vi "Turbo Pump Control.vi"(8 "error in (no error)":errorcluster, 11 "cRIO-CO2 in":refnum<class "cRIO-CO2.lvclass">) -> ()   [LabVIEW 2015, in "cRIO-Carbondioxide.lvlib" / "cRIO-CO2.lvlib" / "cRIO-CO2.lvclass"]
uses:
  cRIO-CO2.lvclass
  <instrlib>/BOC Edwards TIC/Turbo Instrument Controller.llb/Type Def - Pump State.ctl
  <instrlib>/BOC Edwards TIC/Turbo Instrument Controller.llb/Type Def - Alert ID.ctl
  <instrlib>/BOC Edwards TIC/Turbo Instrument Controller.llb/Type Def - Priority.ctl
  Controls/Pumping State Enumerator.ctl
panel:
  in  "Running Dt":i32=1000
  out "Alert Priority":T1
  out "Status":T2
  out "Turbo Pump State":T3
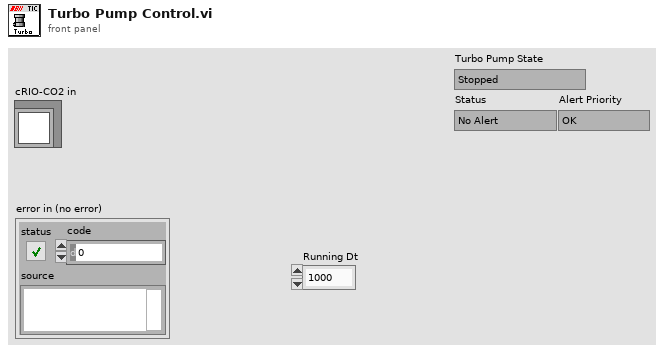
[diagram p1: front panel]
types:
  T1 = typedef "Type Def - Priority.ctl" = enum16{"OK", "Warning", "Alarm"}
  T2 = typedef "Type Def - Alert ID.ctl" = enum16{"No Alert", "ADC Fault", "ADC Not Ready", "Over Range", "Under Range", "ADC Invalid", "No Gauge", "Unknown", "Not Supported", "New ID", "Ion EM Timeout", "Not Struck", "Filament Fail", "Mag Fail", "Striker Fail", "Cal Error", "Initialising", "Emission Error", "Over Pressure", "ASG Can't Zero", "Ramp Up Timeout", "Droop Timeout", "Run Hours High", "SC Interlock", "ID Volts Error", "Serial ID Fail", "Upload Active", "DX Fault", "Temp Alert", "SYSI Inhibit", "Ext Inhibit", "Temp Inhibit", "No Reading", "No Message", "NOV Failure", "ULoad Timeout", "DLoad Failed", "No Tube"}
  T3 = typedef "Type Def - Pump State.ctl" = enum16{"Stopped", "Starting Delay", "Stopping Short Delay", "Stopping Normal Delay", "Running", "Accelerating", "Fault Braking", "Braking"}
  T4 = typedef "Pumping State Enumerator.ctl" = enum16{"Initialize", "Idle", "Error", "Start FV Pump", "Wait on FV Gauge", "Start Turbo", "Running", "Stop"}
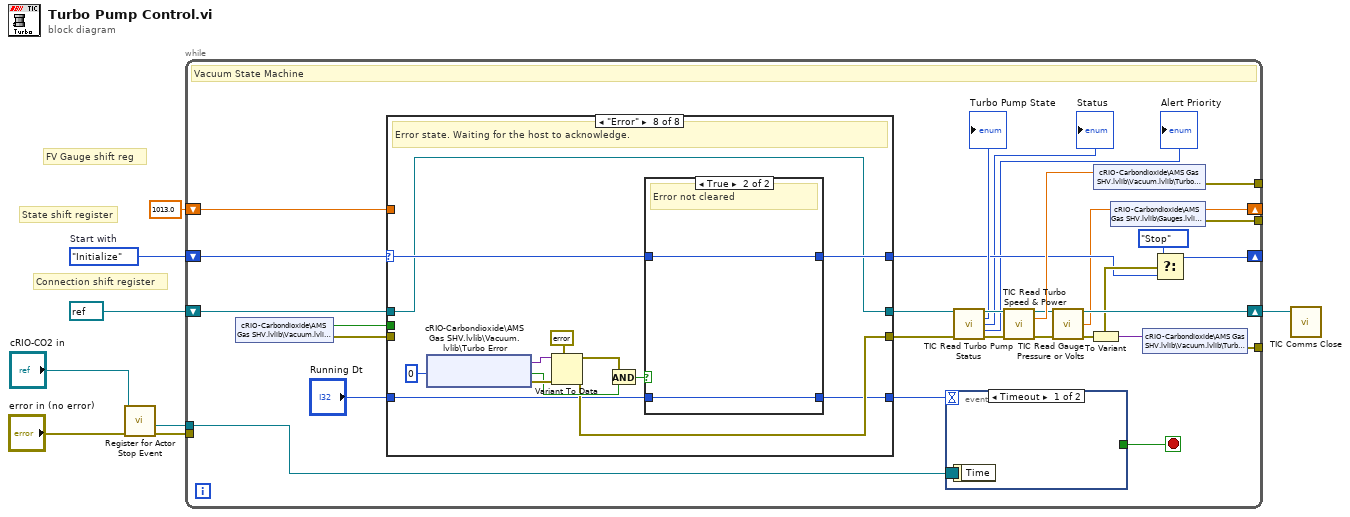
[diagram p0: block diagram]
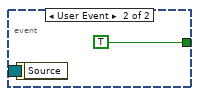
[diagram p2: hidden frame]
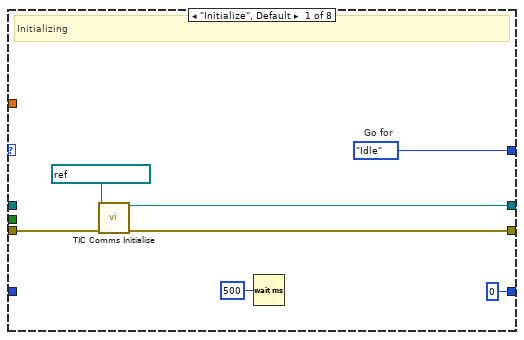
[diagram p3: hidden frame]
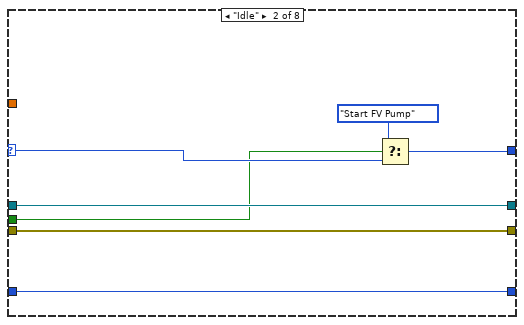
[diagram p4: hidden frame]
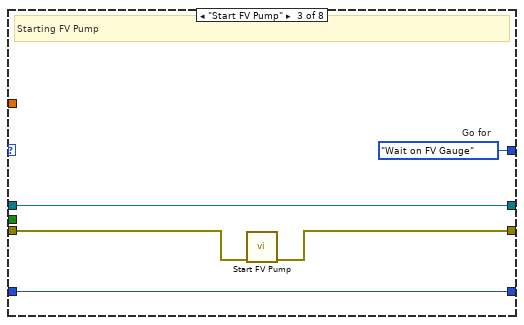
[diagram p5: hidden frame]
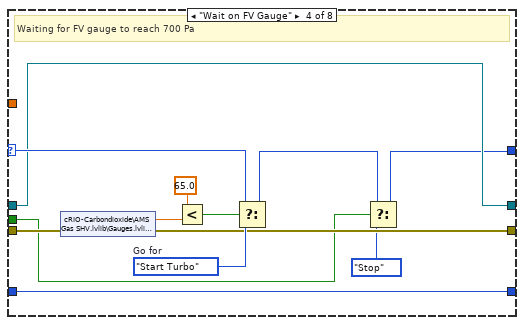
[diagram p6: hidden frame]
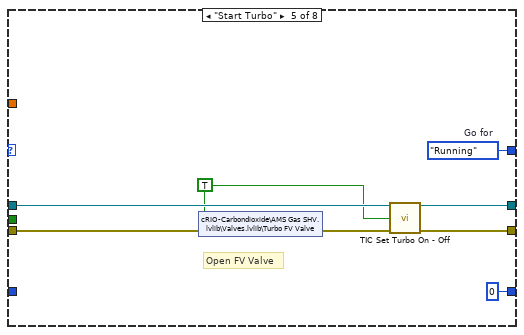
[diagram p7: hidden frame]
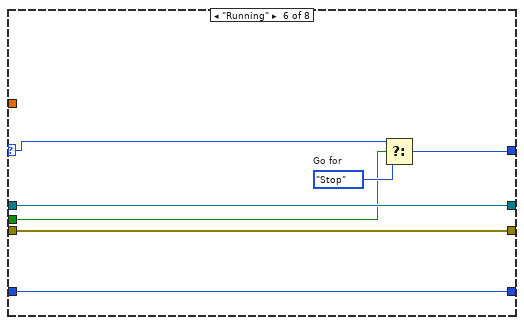
[diagram p8: hidden frame]
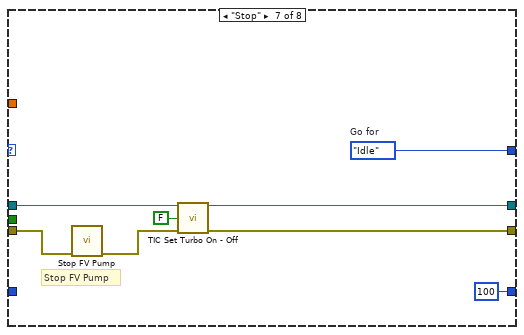
[diagram p9: hidden frame]
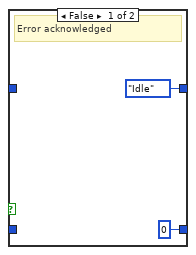
[diagram p10: hidden frame]
diagram:
  w8 = Pumping_State_Enumerator."Initialize"  # Start with
  # "FV Gauge shift reg"
  # "Connection shift register"
  # "State shift register"
  n1 = call "Register for Actor Stop Event.vi"("error in (no error)"="error in (no error)", "cRIO-CO2 in"="cRIO-CO2 in") -> ("error out"=w1:errorcluster, "Event Registration Refnum"=w2:refnum<event-registration>)  [unwired: 7 in, 1 out]
  n2 = while {
    shift-right: [w34] -> w6
    shift-left: refnum<visa-resource-name> refnum ("VISA session (Dup)") -> [w37]
    shift-right: [w22] -> _
    shift-left: w8 -> [w15]
    tunnel: [w35] -> _
    tunnel: [w31] -> _
    tunnel: [w30] -> _
    shift-right: [w14] -> _
    shift-left: 1013.0 ("Reading") -> [w13]
    tunnel: w2 -> [w11]
    tunnel: w1 -> [_]
    stop <- w10 stop-if-true
    # "Vacuum State Machine"
    n3 = shared-variable "cRIO-Carbondioxide\\AMS Gas SHV.lvlib\\Vacuum.lvlib\\Turbo ON"() -> (w16:bool, error out=w23:errorcluster)  [unwired: 1 in]
    n4 = case shown="\"Error\"" w15 {
      selector: w15 -> [_ w50 _ w66 _ w81 _ w99]
      tunnel: [w45 w52 w54 w63 w76 w85 w91 w97] -> w28
      tunnel: w37 -> [_ w52 w54 w63 w77 w85 w86 w97]
      tunnel: [w41 w51 w57 w61 w72 w80 w89 w98] -> w20
      tunnel: [w43 w48 w56 w64 w78 w84 w92 w96] -> w26
      tunnel: [0 w46 w53 w59 0 w79 100 w95] -> w12
      tunnel: w23 -> [w39 w48 w55 w70 w71 w84 w88 _]
      tunnel: w16 -> [_ w47 _ w58 _ w82 _ _]
      tunnel: w13 -> [_ _ _ _ _ _ _ _]
      tunnel: "Running Dt" -> [_ w46 w53 w59 _ w79 _ w94]
      frame "Initialize", Default {
        w41 = Pumping_State_Enumerator."Idle"  # Go for
        # "Initializing"
        n5 = call <instrlib>:"TIC Comms Initialise.vi"("VISA Resource Name"=refnum<visa-resource-name> "ASRL1::INSTR", "error in (no error)"=w39) -> ("VISA session (Dup)"=w45:refnum<visa-resource-name>, "error out"=w43:errorcluster)  [unwired: 12 in]
        n6 = Wait (ms)(milliseconds to wait=u32 500) -> ()  [unwired: 1 out]
      }
      frame "Idle" {
        n7 = Select(t=Pumping_State_Enumerator."Start FV Pump", s=w47, f=w50) -> (s? t:f=w51:T4)
      }
      frame "Start FV Pump" {
        w57 = Pumping_State_Enumerator."Wait on FV Gauge"  # Go for
        # "Starting FV Pump"
        n8 = call "Start FV Pump.vi"("error in (no error)"=w55) -> ("error out"=w56:errorcluster)  [unwired: 10 in]
      }
      frame "Wait on FV Gauge" {
        w65 = Pumping_State_Enumerator."Start Turbo"  # Go for
        # "Waiting for FV gauge to reach 700 Pa"
        n9 = shared-variable "cRIO-Carbondioxide\\AMS Gas SHV.lvlib\\Gauges.lvlib\\FV Gauge"(error in=w70) -> (w69:dbl, error out=w64:errorcluster)
        n10 = Less?(x=65.0, y=w69) -> (x < y?=w67:bool)
        n11 = Select(t=w66, s=w67, f=w65) -> (s? t:f=w62:T4)
        n12 = Select(t=w62, s=w58, f=Pumping_State_Enumerator."Stop") -> (s? t:f=w61:T4)
      }
      frame "Start Turbo" {
        w72 = Pumping_State_Enumerator."Running"  # Go for
        w73 = TRUE ("Turbo FV valve")
        # "Open FV Valve"
        n13 = shared-variable "cRIO-Carbondioxide\\AMS Gas SHV.lvlib\\Valves.lvlib\\Turbo FV Valve"(w73, error in=w71) -> (error out=w74:errorcluster)
        n14 = call <instrlib>:"TIC Set Turbo On - Off.vi"("VISA Session In"=w77, "On (F)"=w73, "error in (no error)"=w74) -> ("VISA Session (Dup)"=w76:refnum<visa-resource-name>, "error out"=w78:errorcluster)  [unwired: 11 in]
      }
      frame "Running" {
        w83 = Pumping_State_Enumerator."Stop"  # Go for
        n15 = Select(t=w81, s=w82, f=w83) -> (s? t:f=w80:T4)
      }
      frame "Stop" {
        w89 = Pumping_State_Enumerator."Idle"  # Go for
        # "Stop FV Pump"
        n16 = call "Stop FV Pump.vi"("error in (no error)"=w88) -> ("error out"=w87:errorcluster)  [unwired: 10 in]
        n17 = call <instrlib>:"TIC Set Turbo On - Off.vi"("VISA Session In"=w86, "On (F)"=FALSE, "error in (no error)"=w87) -> ("VISA Session (Dup)"=w91:refnum<visa-resource-name>, "error out"=w92:errorcluster)  [unwired: 11 in]
      }
      frame "Error" {
        # "Error state. Waiting for the host to acknowledge."
        n18 = shared-variable "cRIO-Carbondioxide\\AMS Gas SHV.lvlib\\Vacuum.lvlib\\Turbo Error"(0 ("ms timeout (0)")) -> (w103:variant, error out=w104:errorcluster, w100:bool)  [unwired: 1 in]
        n19 = Variant To Data(error in=w104, type=errorcluster {"status"=FALSE, "code"=0, "source"=""} ("error out"), Variant=w103) -> (data=w101:errorcluster, error out=w96:errorcluster)
        n20 = And(x=w101, y=w100) -> (x .and. y?=w105:bool)
        n21 = case shown="True" w105 {
          tunnel: w99 -> [_ w110]
          tunnel: [Pumping_State_Enumerator."Idle" w110] -> w98
          tunnel: [0 w109] -> w95
          tunnel: w94 -> [_ w109]
          frame False {
            # "Error acknowledged"
          }
          frame True {
            # "Error not cleared"
          }
        }
      }
    }
    n22 = event shown="[0] Timeout" {
      selector: w11 -> [_ _]
      dyn-events: _ -> [_ _]
      timeout: w12 -> [_ _]
      tunnel: [_ TRUE] -> w10
      event Timeout {
        n23 = event-data() -> ()  [unwired: 1 in, 1 out]
      }
      event User Event {
        n24 = event-data() -> ()  [unwired: 1 in, 1 out]
      }
    }
    n25 = call <instrlib>:"TIC Read Turbo Pump Status.vi"("VISA Resource Name"=w28, "error in (no error)"=w26) -> ("VISA session (Dup)"=w27:refnum<visa-resource-name>, "Turbo Pump State"=→"Turbo Pump State":T3, "Status"=→"Status":T2, "Alert Priority"=→"Alert Priority":T1, "error out"=w25:errorcluster)  [unwired: 9 in]
    n26 = call <instrlib>:"TIC Read Turbo Speed & Power.vi"("VISA Resource Name"=w27, "error in (no error)"=w25) -> ("VISA session (Dup)"=w29:refnum<visa-resource-name>, "Pump Speed (%)"=w32:dbl, "error out"=w33:errorcluster)  [unwired: 9 in, 2 out]
    n27 = call <instrlib>:"TIC Read Gauge Pressure or Volts.vi"("VISA Session In"=w29, "error in (no error)"=w33) -> ("VISA Session (Dup)"=w34:refnum<visa-resource-name>, "Reading"=w14:dbl, "error out"=w21:errorcluster)  [unwired: 9 in, 2 out]
    n28 = To Variant(anything=w21) -> (Variant=w36:variant)
    n29 = shared-variable "cRIO-Carbondioxide\\AMS Gas SHV.lvlib\\Vacuum.lvlib\\Turbo Speed"(w32) -> (error out=w31:errorcluster)  [unwired: 1 in]
    n30 = shared-variable "cRIO-Carbondioxide\\AMS Gas SHV.lvlib\\Gauges.lvlib\\FV Gauge"(w14) -> (error out=w30:errorcluster)  [unwired: 1 in]
    n31 = shared-variable "cRIO-Carbondioxide\\AMS Gas SHV.lvlib\\Vacuum.lvlib\\Turbo Error"(w36) -> (error out=w35:errorcluster)  [unwired: 1 in]
    n32 = Select(t=Pumping_State_Enumerator."Stop", s=w21, f=w20) -> (s? t:f=w22:T4)
  }
  n33 = call <instrlib>:"TIC Comms Close.vi"("VISA Resource Name"=w6) -> ()  [unwired: 14 in, 1 out]
